vi "GetDataEventStreamProperties.vi"(11 "data event":T1) -> (0 "last block":bool, 1 "block":i32, 2 "stream Id":string, 3 "stream":bool)   [LabVIEW 2017, in "DataEvent.lvlib"]
uses:
  <vilib>/addons/InsightCM/Devices/Shared/Common/DataEvent/DataEvent.lvlib
  <vilib>/addons/InsightCM/Devices/Shared/Common/DataEvent/controls/Event.ctl
  <vilib>/addons/InsightCM/MessageBus/Base/controls/DataEvent.ctl
  <vilib>/addons/InsightCM/MessageBus/Base/controls/KeyValuePair.ctl
  <vilib>/addons/InsightCM/Devices/Shared/Common/DataEvent/controls/DataSet.ctl
  <vilib>/addons/InsightCM/MessageBus/Base/controls/DataSetMetadata.ctl
  <vilib>/addons/InsightCM/MessageBus/Base/controls/TrendPoint.ctl
  <vilib>/addons/InsightCM/MessageBus/Base/controls/TrendAlarmUpdate.ctl
  <vilib>/addons/InsightCM/MessageBus/Base/controls/TrendAlarmTransition.ctl
  <vilib>/addons/InsightCM/Utilities/PropertyHelpers/PropertyHelpers.lvlib
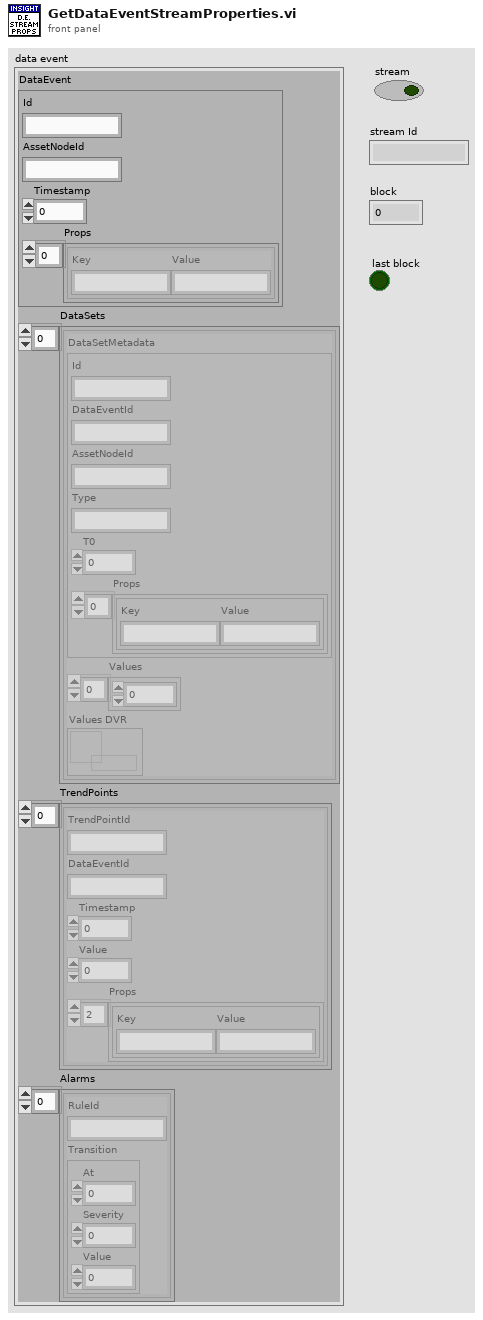
[diagram p1: front panel]
types:
  T1 = typedef "DataEvent.lvlib/Event.ctl" = cluster{"DataEvent":T2, "DataSets":T4[], "TrendPoints":T6[], "Alarms":T7[]}
  T2 = typedef "DataEvent.ctl" = cluster{"Id":string, "AssetNodeId":string, "Timestamp":i64, "Props":T3[]}
  T3 = typedef "KeyValuePair.ctl" = cluster{"Key":string, "Value":string}
  T4 = typedef "DataEvent.lvlib/DataSet.ctl" = cluster{"DataSetMetadata":T5, "Values":sgl[], "Values DVR":refnum<data-value>}
  T5 = typedef "DataSetMetadata.ctl" = cluster{"Id":string, "DataEventId":string, "AssetNodeId":string, "Type":string, "T0":i64, "Props":T3[]}
  T6 = typedef "TrendPoint.ctl" = cluster{"TrendPointId":string, "DataEventId":string, "Timestamp":i64, "Value":dbl, "Props":T3[]}
  T7 = typedef "TrendAlarmUpdate.ctl" = cluster{"RuleId":string, "Transition":T8}
  T8 = typedef "TrendAlarmTransition.ctl" = cluster{"At":i64, "Severity":i32, "Value":dbl}
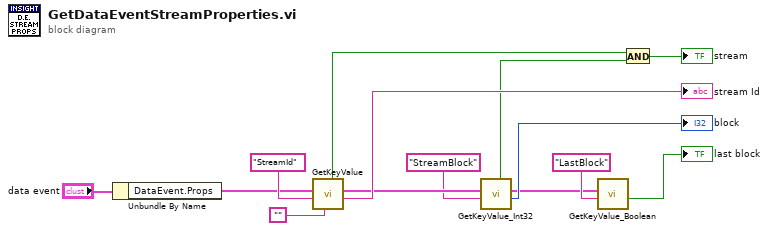
[diagram p0: block diagram]
diagram:
  n1 = Unbundle By Name("data event") -> ("DataEvent.Props"=w12:T3[])
  n2 = call <vilib>:"GetKeyValue.vi"("default value"="", "key"="StreamId", "key value pairs"=w12) -> ("value"=→"stream Id":string, "key value pairs out"=w9:T3[], "found"=w2:bool)  [unwired: 6 in]
  n3 = call <vilib>:"GetKeyValue_Int32.vi"("key"="StreamBlock", "key value pairs"=w9) -> ("value"=→"block":i32, "key value pairs out"=w5:T3[], "found"=w3:bool)  [unwired: 7 in]
  n4 = call <vilib>:"GetKeyValue_Boolean.vi"("key"="LastBlock", "key value pairs"=w5) -> ("value"=→"last block":bool)  [unwired: 7 in, 2 out]
  n5 = And(x=w2, y=w3) -> (x .and. y?=→"stream":bool)
